vi "DragDropMoveCopyFindParent.vi"(5 "ParentChild":cluster{"Parent":i32, "Child":i32}, 7 "Allowed Parent Child":set{cluster{"Parent":i32, "Child":i32}}(c389), 8 "error in (no error)":errorcluster, 9 "InBounds":bool, 10 "Drag Status":T1, 11 "TreeControl in":refnum<vi>) -> (0 "error out":errorcluster, 1 "Insert Inex":i32, 2 "Parent Tag":string, 3 "TreeControl out":refnum<vi>)   [LabVIEW 2019, in "TreeControlLib.lvlib"]
uses:
  TreeControlLib.lvlib
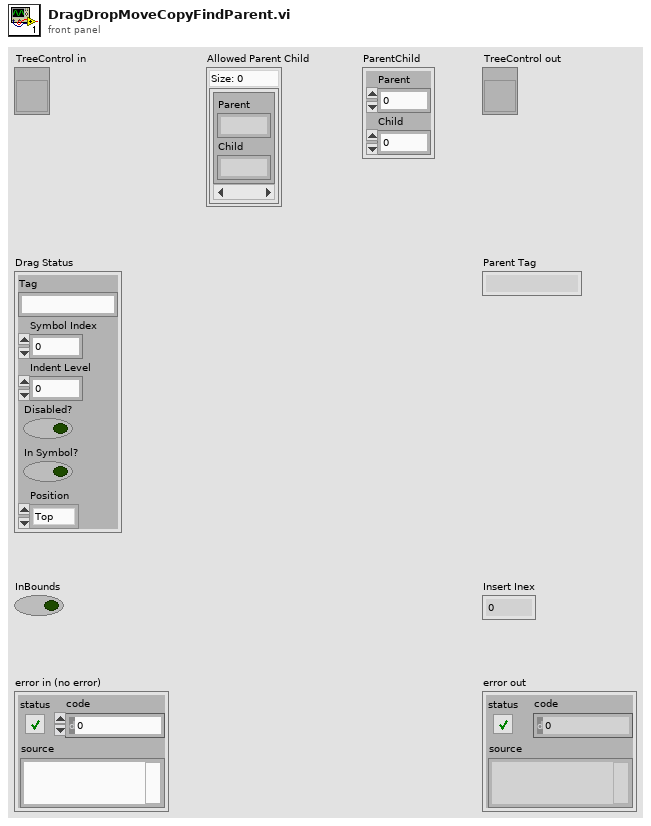
[diagram p1: front panel]
types:
  T1 = cluster{"Tag":string, "Symbol Index":i32, "Indent Level":i32, "Disabled?":bool, "In Symbol?":bool, "Position":enum16{"Top", "Center", "Bottom"}}
  T2 = enum16{"FirstChild", "PreviousSibling", "NextSibling"}
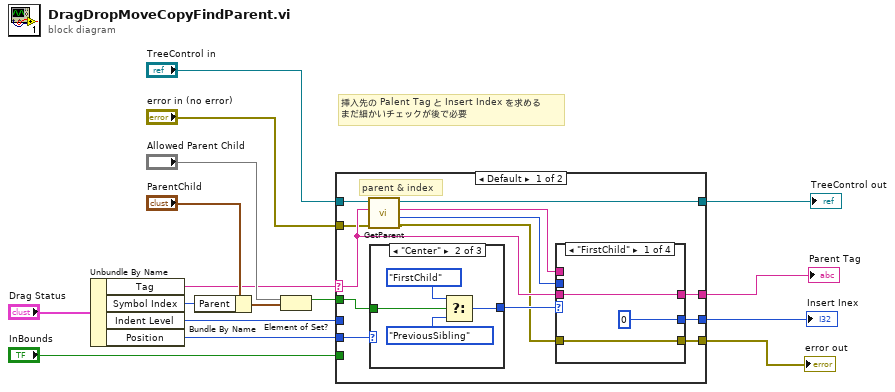
[diagram p0: block diagram]
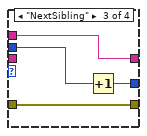
[diagram p3: hidden frame]
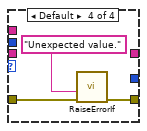
[diagram p4: hidden frame]
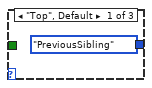
[diagram p5: hidden frame]
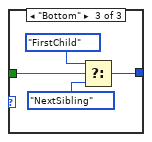
[diagram p6: hidden frame]
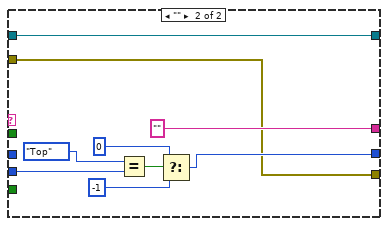
[diagram p7: hidden frame]
diagram:
  # "挿入先の Palent Tag と Insert Index を求める\nまだ細かいチェックが後で必要"
  n1 = Unbundle By Name("Drag Status") -> ("Tag"=w4:string, "Symbol Index"=w7:i32, "Indent Level"=w2:i32, "Position"=w1:enum16{"Top", "Center", "Bottom"})
  n2 = Bundle By Name(cluster="ParentChild", "Parent"=w7) -> (w10:cluster{"Parent":i32, "Child":i32})
  n3 = Element of Set?(10:w10, 11:"Allowed Parent Child") -> (3:w8:bool)
  n4 = case shown="Default" w4 {
    selector: w4 -> [w26 _]
    tunnel: "InBounds" -> [_ _]
    tunnel: w2 -> [_ _]
    tunnel: w1 -> [w29 w60]
    tunnel: "TreeControl in" -> [w28 w52]
    tunnel: [w25 w55] -> w6
    tunnel: [w24 "" ("Parent Tag")] -> w13
    tunnel: w8 -> [w23 _]
    tunnel: "error in (no error)" -> [w22 w53]
    tunnel: [w20 w53] -> w11
    tunnel: [w17 w52] -> w16
    frame Default {
      # "parent & index"
      n5 = call "GetParent.vi"("error in (no error)"=w22, "Tag"=w26, "TreeControl in"=w28) -> ("error out"=w21:errorcluster, "Child Index"=w19:i32, "Parent Tag"=w18:string, "TreeControl out"=w17:refnum<vi>)  [unwired: 5 in]
      n6 = case shown="\"Center\"" w29 {
        tunnel: w23 -> [_ w46 w50]
        tunnel: [T2."PreviousSibling" w44 w48] -> w27
        frame "Top", Default {
        }
        frame "Center" {
          n7 = Select(t=T2."FirstChild", s=w46, f=T2."PreviousSibling") -> (s? t:f=w44:T2)
        }
        frame "Bottom" {
          n8 = Select(t=T2."FirstChild", s=w50, f=T2."NextSibling") -> (s? t:f=w48:T2)
        }
      }
      n9 = case shown="\"FirstChild\"" w27 {
        tunnel: w18 -> [_ w35 w39 _]
        tunnel: w19 -> [_ w34 w38 _]
        tunnel: w26 -> [w32 _ _ _]
        tunnel: [w32 w35 w39 _] -> w24
        tunnel: [0 w34 w37 _] -> w25
        tunnel: w21 -> [w30 w33 w36 w41]
        tunnel: [w30 w33 w36 w40] -> w20
        frame "FirstChild" {
        }
        frame "PreviousSibling" {
        }
        frame "NextSibling" {
          n10 = Increment(x=w38) -> (x+1=w37:i32)
        }
        frame Default {
          n11 = call "RaiseErrorIf.vi"("error in (no error)"=w41, "error message"="Unexpected value.") -> ("error out"=w40:errorcluster)  [unwired: 9 in]
        }
      }
    }
    frame "" {
      n12 = Equal?(x=enum16{"Top", "Center", "Bottom"}."Top", y=w60) -> (x = y?=w58:bool)
      n13 = Select(t=0, s=w58, f=-1) -> (s? t:f=w55:i32)
    }
  }
  "TreeControl out" <- w16
  "Parent Tag" <- w13
  "error out" <- w11
  "Insert Inex" <- w6
